vi "Stop Core.vi"(10 "final error code":i32, 11 "CS++GoBangServer in":refnum<class "CS++GoBangServer.lvclass">) -> (3 "CS++GoBangServer out":refnum<class "CS++GoBangServer.lvclass">)   [LabVIEW 2014, in "GoBang.lvlib" / "CS++GoBangServer.lvclass"]
doc: "(<B>Filename</B>: Actor Framework.lvlib:Actor.lvclass:Stop Core.vi)\n\nDefines what the actor does before it stops. Use the <B>final error code</B> input to determine whether the actor shut down in response to an error.\n\nBy default, this method does nothing. A descendant class may override it to define behavior, such as shutting down any processes the actor initiated in its override of the Actor Core method."
uses:
  CS++GoBangServer.lvclass
  CS++GoBangServer.lvclass/CS++GoBangServer.ctl
  <vilib>/ActorFramework/Message Enqueuer/Message Enqueuer.lvclass/Message Enqueuer.ctl
  <vilib>/ActorFramework/Message Enqueuer/Enqueue.vi
  <vilib>/ActorFramework/Message Priority Queue/Priority Enqueue.vi
  CSPP_Core/Actors/CS++BaseActor/CS++BaseActor.lvclass
  <vilib>/ActorFramework/Stop Msg/Stop Msg.lvclass
  CSPP_Core/Classes/CS++ProcessVariables/PVConnection/PVConnection.lvclass
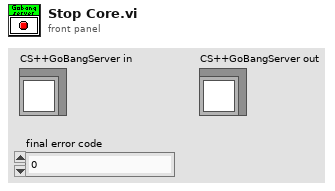
[diagram p1: front panel]
types:
  T1 = cluster{"BlackPlayer":refnum<class "PVConnection.lvclass">, "WhitePlayer":refnum<class "PVConnection.lvclass">, "GameBoard":refnum<class "PVConnection.lvclass">, "GameState":refnum<class "PVConnection.lvclass">}
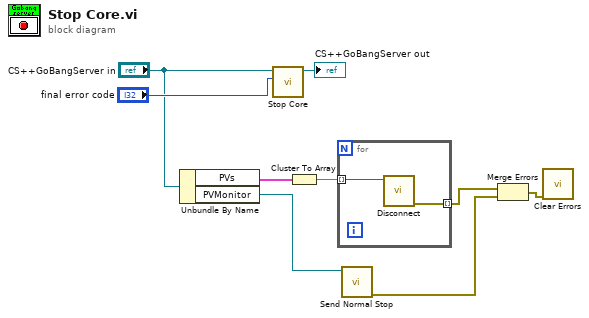
[diagram p0: block diagram]
diagram:
  n1 = Unbundle By Name("CS++GoBangServer in") -> ("PVs"=w6:T1, "PVMonitor"=w4:refnum<class "Message Enqueuer.lvclass">)
  n2 = call-parent "Stop Core.vi"("final error code"="final error code", "CS++BaseActor in"="CS++GoBangServer in") -> ("CS++BaseActor out"=→"CS++GoBangServer out":refnum<class "CS++GoBangServer.lvclass">)  [unwired: 9 in]
  n3 = Cluster To Array(cluster=w6) -> (array=w5:refnum<class "PVConnection.lvclass">[])
  n4 = for {
    tunnel: w5 -> [w11] mode=indexing
    tunnel: [w10] -> w2 mode=indexing
    n5 = call "Disconnect.vi"("PVConnection in"=w11) -> ("error out"=w10:errorcluster)  [unwired: 9 in, 1 out]
  }
  n6 = call <vilib>:"Send Normal Stop.vi"("Message Enqueuer"=w4) -> ("error out"=w3:errorcluster)  [unwired: 10 in]
  n7 = Merge Errors(w2, w3) -> (w1:errorcluster)
  n8 = call <vilib>:"Clear Errors.vi"("error in (no error)"=w1) -> ()  [unwired: 5 in, 2 out]
